vi "load_data.vi"(0 "datasource_webpage in":refnum<class "datasource_webpage.lvclass">, 11 "error in (no error)":errorcluster) -> (4 "datasource_webpage out":refnum<class "datasource_webpage.lvclass">, 6 "document":refnum<class "data_document.lvclass">[](array[class]), 15 "error out":errorcluster)   [LabVIEW 2020, in "datasource_webpage.lvclass"]
uses:
  datasource_webpage.lvclass
  data/data_document/data_document.lvclass
  datasource_webpage.lvclass/datasource_webpage.ctl
  <vilib>/httpClient/LabVIEWHTTPClient.lvlib
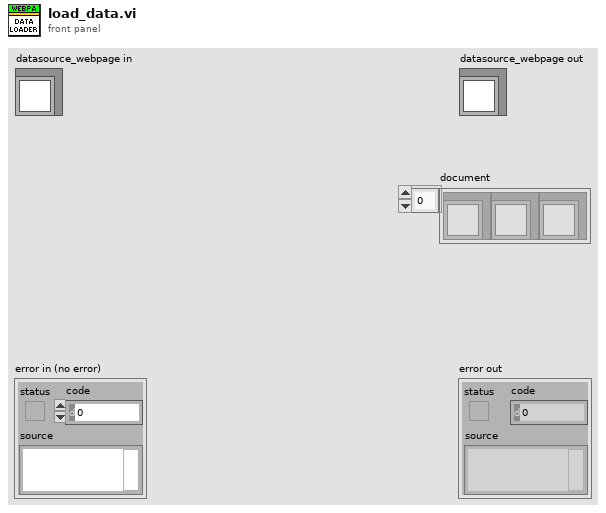
[diagram p1: front panel]
types:
  T1 = typedef "LabVIEWHTTPClient.lvlib/ClientHandle.ctl" = refnum<k1>
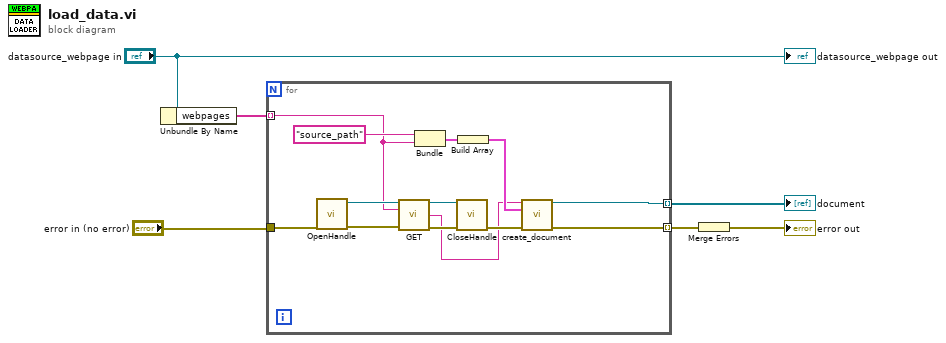
[diagram p0: block diagram]
diagram:
  n1 = Unbundle By Name("datasource_webpage in") -> ("webpages"=w2:string[])
  n2 = for {
    tunnel: [w15] -> w4 mode=indexing
    tunnel: w2 -> [w8] mode=indexing
    tunnel: "error in (no error)" -> [w12]
    tunnel: [w16] -> w5 mode=indexing
    n3 = call <vilib>:"OpenHandle.vi"("error in (no error)"=w12) -> ("client handle out"=w13:T1, "error out"=w14:errorcluster)  [unwired: 13 in]
    n4 = call <vilib>:"GET.vi"("client handle"=w13, "url"=w8, "error in (no error)"=w14) -> ("client handle out"=w9:T1, "body"=w7:string, "error out"=w11:errorcluster)  [unwired: 9 in, 1 out]
    n5 = Bundle("source_path", "String"=w8) -> (w18:cluster{string, "String":string})  [unwired: 1 in]
    n6 = call <vilib>:"CloseHandle.vi"("client handle"=w9, "error in (no error)"=w11) -> ("error out"=w10:errorcluster)  [unwired: 13 in]
    n7 = Build Array(w18) -> (w17:cluster{string, "String":string}[])
    n8 = call "create_document.vi"("text"=w7, "metadatas"=w17, "error in (no error)"=w10) -> ("data_document out"=w15:refnum<class "data_document.lvclass">, "error out"=w16:errorcluster)  [unwired: 11 in]
  }
  "document" <- w4
  n9 = Merge Errors(w5) -> (→"error out":errorcluster)
  "datasource_webpage out" <- "datasource_webpage in"
